vi "Beacon_Filtering_Inter_Beacon_Distance_R1.vi"(0 "Num of Beacons":i8=5, 1 "Inter Beacon\nReal Distance":sgl=3.0, 5 "X in":sgl[](array[numeric]), 7 "Inter Beacon\ndelta Threshold":sgl=1.0, 9 "Y in":sgl[](array[numeric]), 11 "Valid Data\nSets in":bool[](array[boolean])=[TRUE, TRUE, TRUE, TRUE, TRUE]) -> (4 "Beacons Valid - Out":bool[](array[boolean]))   [LabVIEW 2015]
panel:
  in  "Intercept":sgl format="%#_13g"
  in  "Slope":sgl format="%#_13g"
  out "Debug Inter DIstances":sgl[][](array[numeric])
  out "Debug Out\nDistances":sgl[][](array[numeric])
  out "Debug Out\nP/F for each\nanchor":bool[][](array[boolean])
  # "INPUTS"
  # "CONFIG"
  # "OUTPUTS"
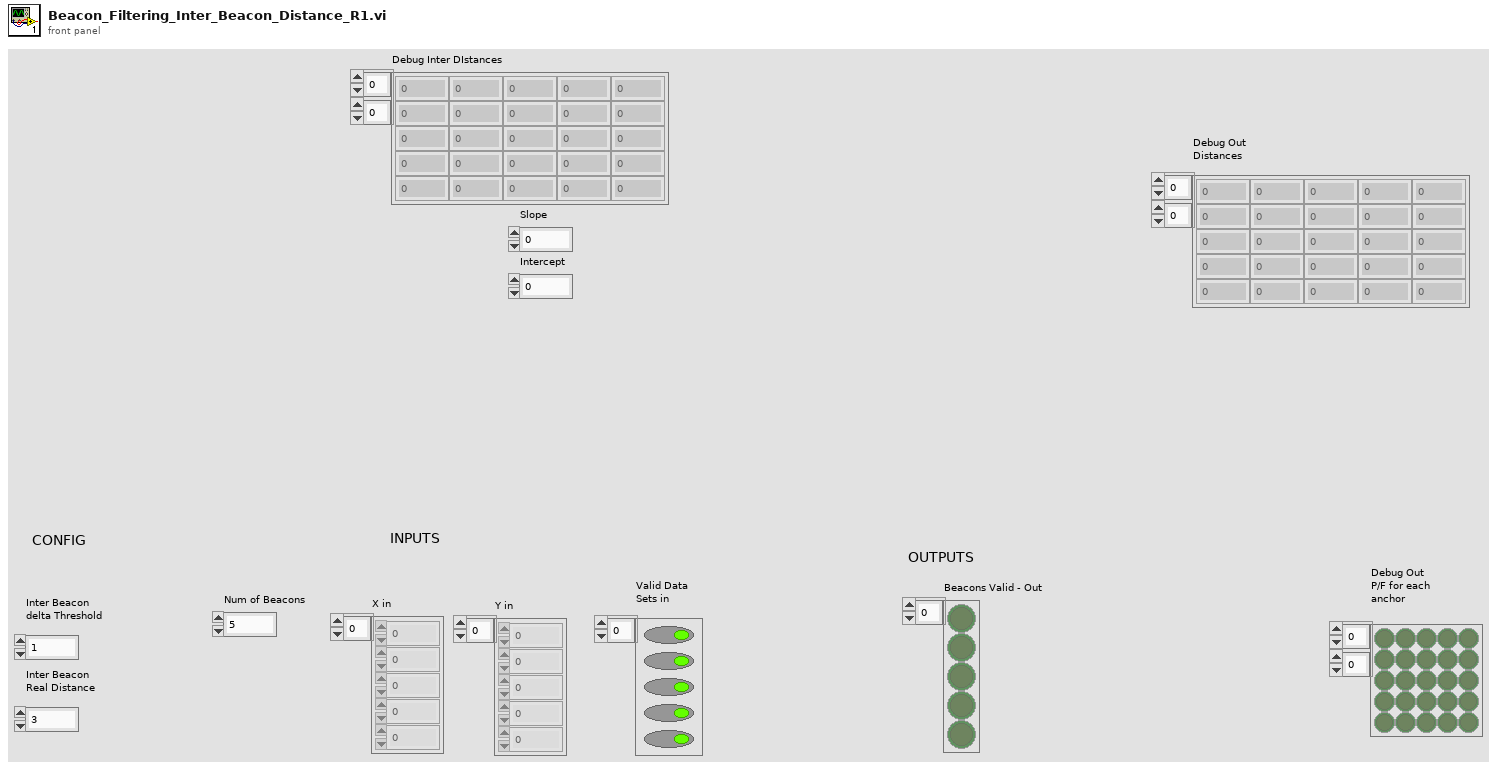
[diagram p1: front panel]
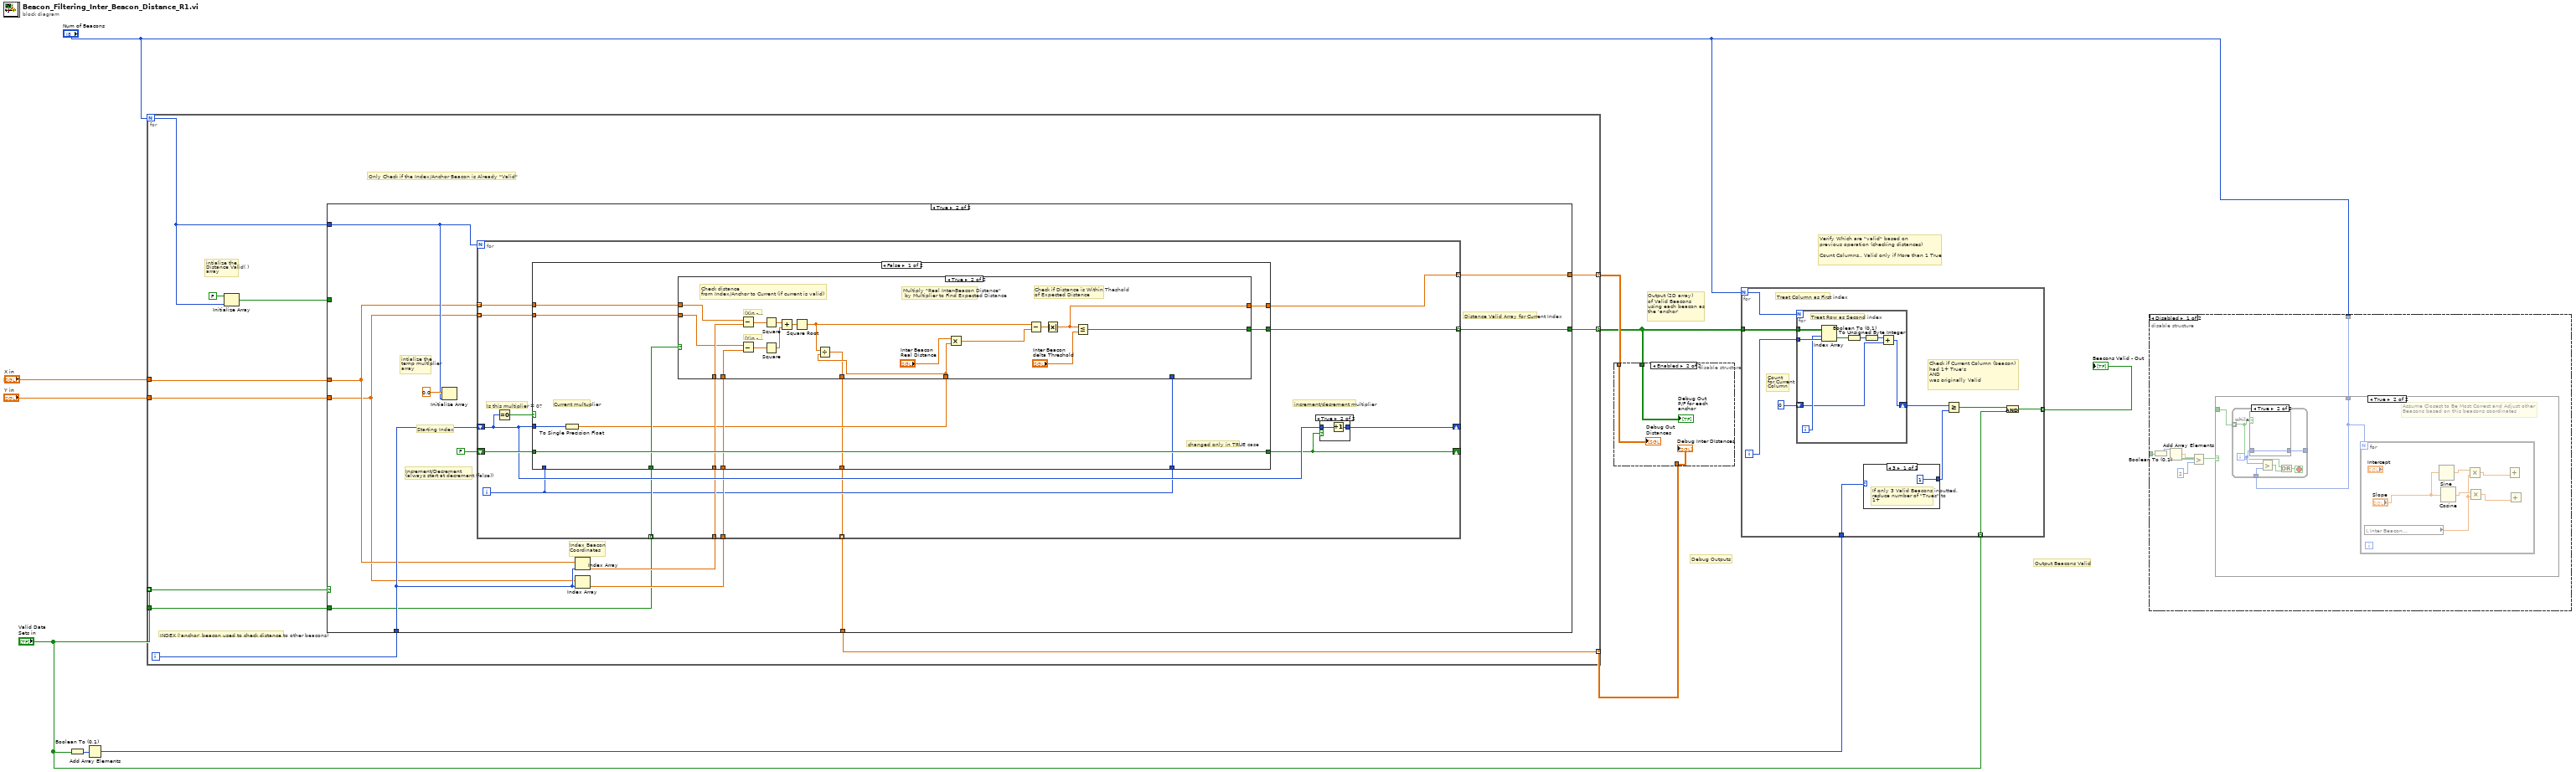
[diagram p0: block diagram]
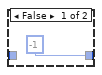
[diagram p3: hidden frame]
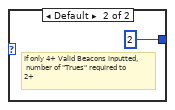
[diagram p6: hidden frame]
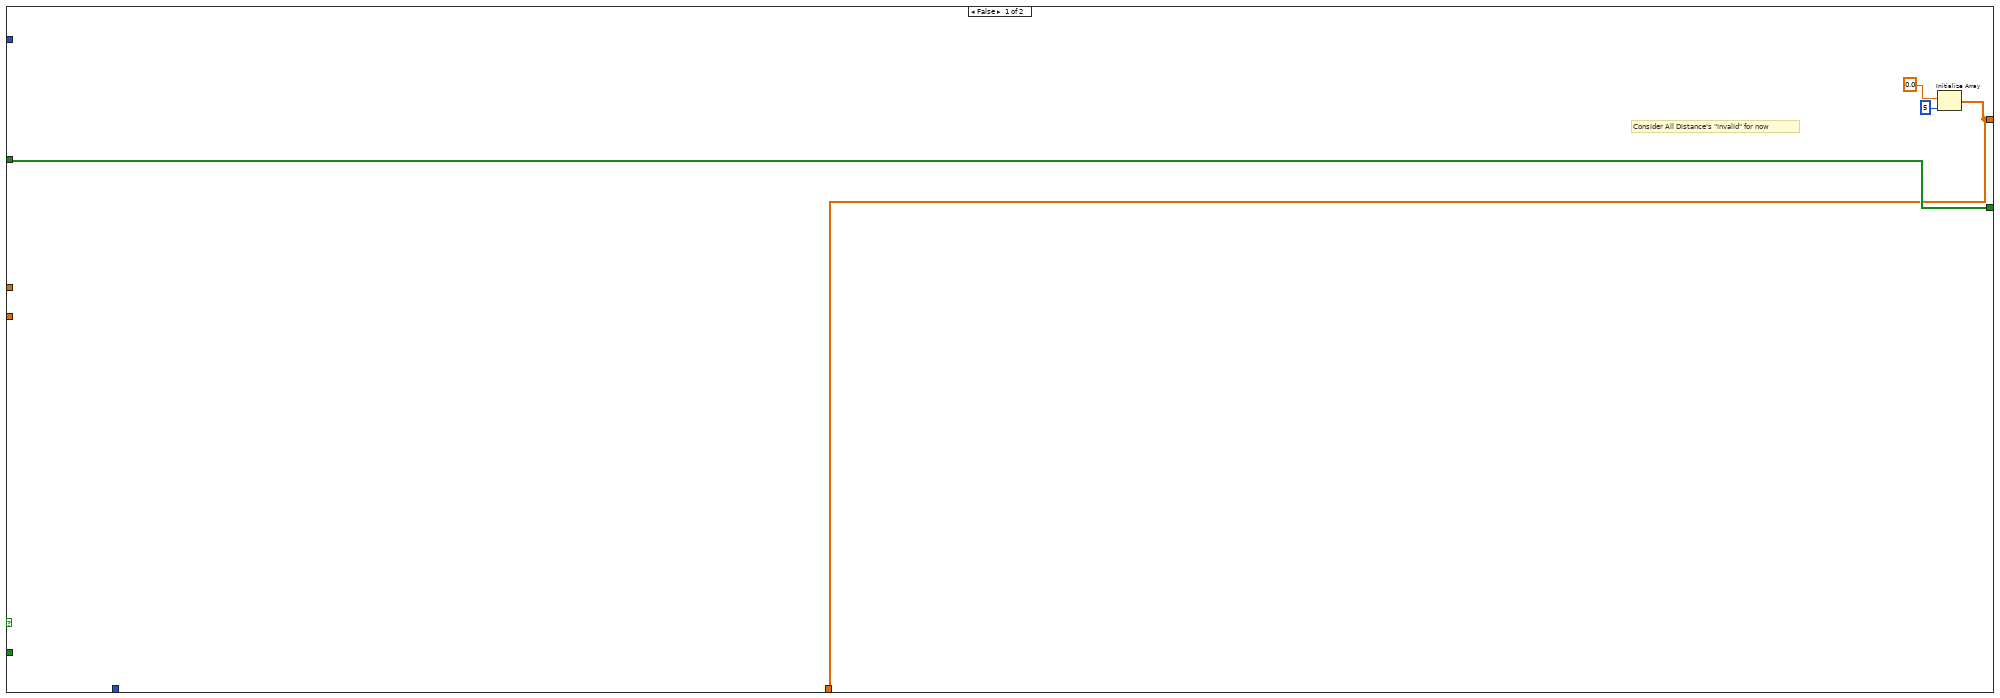
[diagram p7: hidden frame]
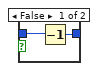
[diagram p8: hidden frame]
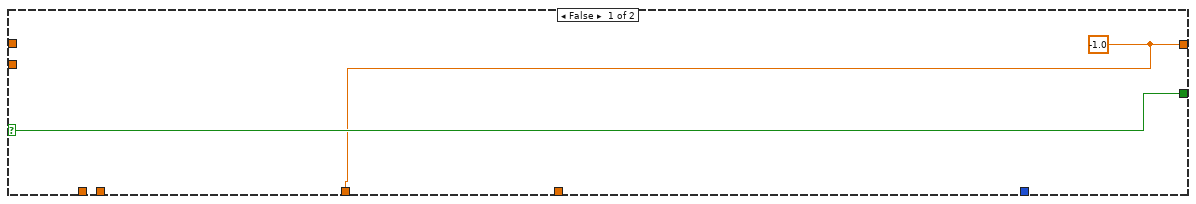
[diagram p9: hidden frame]
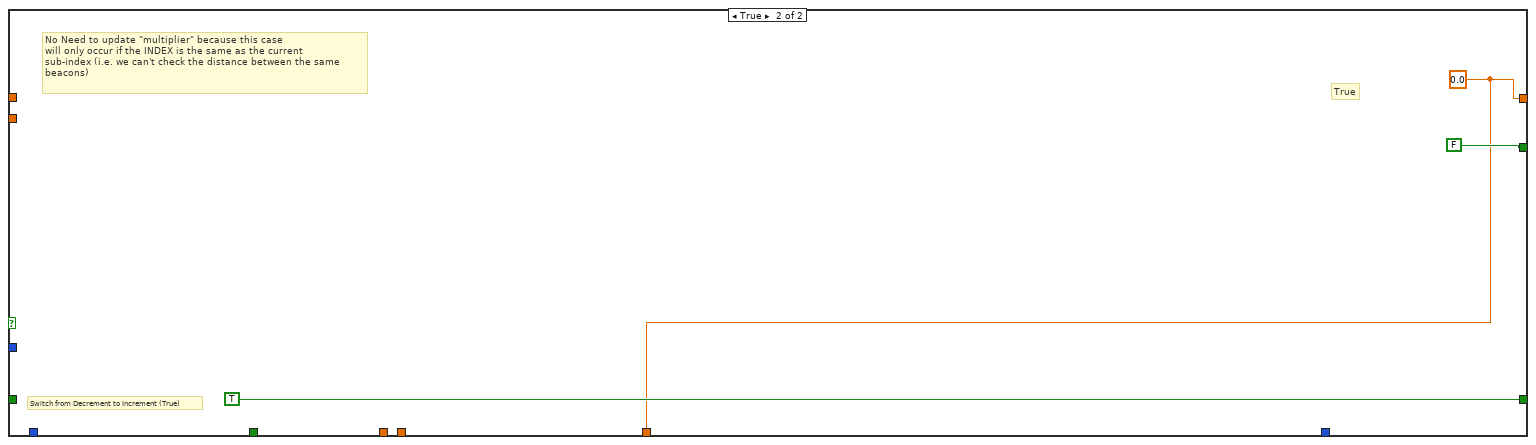
[diagram p10: hidden frame]
diagram:
  # "Debug Outputs"
  # "Output Beacons Valid"
  # "Verify Which are \"valid\" based on \nprevious operation (checking distances)\n\nCount Columns.. Valid only if More than 1 True"
  # "Output (2D array)\nof Valid Beacons\nusing each beacon as\nthe 'anchor'"
  n1 = Boolean To (0,1)(Boolean="Valid Data\nSets in") -> (0, 1=w3:i16[])
  n2 = Add Array Elements(numeric array=w3) -> (sum=w1:i16)
  n3 = for {
    N: "Num of Beacons" -> [w16]
    tunnel: "Valid Data\nSets in" -> [w21] mode=indexing
    tunnel: "X in" -> [w11]
    tunnel: "Y in" -> [w20]
    tunnel: "Valid Data\nSets in" -> [w18]
    tunnel: [w14] -> w4 mode=indexing
    tunnel: [w13] -> w10 mode=indexing
    tunnel: [w12] -> w9 mode=indexing
    i -> [w19]
    # "intialize the \nDistance Valid( )\narray"
    # "INDEX ('anchor' beacon used to check distance to other beacons)"
    # "Only Check if the Index/Anchor Beacon is Already \"Valid\""
    n4 = Initialize Array(FALSE, w16) -> (w15:bool[])
    n5 = case shown="True" w21 {
      tunnel: w11 -> [_ w31]
      tunnel: w20 -> [_ w30]
      tunnel: w19 -> [_ w35]
      tunnel: w16 -> [_ w34]
      tunnel: w18 -> [_ w29]
      tunnel: w15 -> [w25 _]
      tunnel: [w25 w28] -> w14
      tunnel: [w22 w27] -> w13
      tunnel: [w22 w26] -> w12
      frame False {
        # "Consider All Distance's \"invalid\" for now"
        n6 = Initialize Array(sgl 0.0, 5 ("dimension size")) -> (w22:sgl[])
      }
      frame True {
        # "Distance Valid Array for Current Index"
        # "intialize the \ntemp multlplier\narray"
        # "Increment/Decrement\n(always start at decrement (false))"
        # "Starting Index"
        # "Index Beacon\nCoordinates"
        n7 = Initialize Array(sgl 0.0, w34) -> ()  [unwired: 1 out]
        n8 = Index Array(array=w30, index=w35) -> (element=w32:sgl)
        n9 = Index Array(array=w31, index=w35) -> (element=w33:sgl)
        n10 = for {
          N: w34 -> [_]
          shift-right: [w47] -> _
          shift-left: w35 -> [w49]
          shift-right: [w48] -> _
          shift-left: FALSE -> [w50]
          tunnel: w33 -> [w46]
          tunnel: w32 -> [w45]
          tunnel: w31 -> [w44] mode=indexing
          tunnel: w30 -> [w43] mode=indexing
          tunnel: w29 -> [w42] mode=indexing
          tunnel: [w41] -> w28 mode=indexing
          tunnel: [w39] -> w27 mode=indexing
          tunnel: [w38] -> w26 mode=indexing
          i -> [w40]
          # "increment/decrement multiplier"
          # "Is this multiplier = 0?"
          n11 = Equal To 0?(x=w49) -> (x = 0?=w51:bool)
          n12 = case shown="False" w51 {
            tunnel: w49 -> [w67 _]
            tunnel: w40 -> [_ _]
            tunnel: w50 -> [w66 _]
            tunnel: [w66 TRUE] -> w48
            tunnel: w46 -> [w65 _]
            tunnel: w45 -> [w64 _]
            tunnel: w44 -> [w63 _]
            tunnel: w43 -> [w62 _]
            tunnel: w42 -> [w61 _]
            tunnel: [w59 FALSE] -> w41
            tunnel: w40 -> [w58 _]
            tunnel: [w57 w88] -> w39
            tunnel: [w56 w88] -> w38
            frame False {
              # "Current multuplier"
              # "changed only in TRUE case"
              n13 = To Single Precision Float(number=w67) -> (single precision float=w60:sgl)
              n14 = case shown="True" w61 {
                selector: w61 -> [w69 _]
                tunnel: w65 -> [_ w82]
                tunnel: w64 -> [_ w81]
                tunnel: w63 -> [_ w80]
                tunnel: w62 -> [_ w79]
                tunnel: w60 -> [_ w71]
                tunnel: [w69 w74] -> w59
                tunnel: w58 -> [_ _]
                tunnel: [w68 w73] -> w57
                tunnel: [w68 w70] -> w56
                frame False {
                  w68 = sgl -1.0
                }
                frame True {
                  # "Check if Distance is Within Theshold\nof Expected Distance"
                  # "Multiply \"Real Inter-Beacon Distance\"\n by Multiplier to Find Expected Distance"
                  # "(Yin - Y')^2"
                  # "(Xin - X')^2"
                  # "Check distance\nfrom Index/Anchor to Current (if current is valid)"
                  n15 = Subtract(x=w80, y=w82) -> (x-y=w84:sgl)
                  n16 = Subtract(x=w79, y=w81) -> (x-y=w85:sgl)
                  n17 = Square(x=w84) -> (x^2=w86:sgl)
                  n18 = Square(x=w85) -> (x^2=w87:sgl)
                  n19 = Add(x=w86, y=w87) -> (x+y=w83:sgl)
                  n20 = Square Root(x=w83) -> (sqrt(x)=w72:sgl)
                  n21 = Divide(x=w72, y=w71) -> (x/y=w70:sgl)
                  n22 = Multiply(x="Inter Beacon\nReal Distance", y=w71) -> (x*y=w77:sgl)
                  n23 = Subtract(x=w72, y=w77) -> (x-y=w76:sgl)
                  n24 = Absolute Value(x=w76) -> (abs(x)=w73:sgl)
                  n25 = Less Or Equal?(x=w73, y="Inter Beacon\ndelta Threshold") -> (x <= y?=w74:bool)
                }
              }
            }
            frame True {
              w88 = sgl 0.0
              # "True"
              # "Switch from Decrement to Increment (True)"
              # "No Need to update \"multiplier\" because this case\nwill only occur if the INDEX is the same as the current \nsub-index (i.e. we can't check the distance between the same\nbeacons)"
            }
          }
          n26 = case shown="True" w48 {
            tunnel: w49 -> [w53 w55]
            tunnel: [w52 w54] -> w47
            frame False {
              n27 = Decrement(x=w53) -> (x-1=w52:i32)
            }
            frame True {
              n28 = Increment(x=w55) -> (x+1=w54:i32)
            }
          }
        }
      }
    }
  }
  n29 = disable-structure shown="Enabled" {
    disable-tunnel: w4 -> [_ w92]
    disable-tunnel: w10 -> [_ w93]
    disable-tunnel: w9 -> [_ w91]
    frame Disabled {
    }
    frame Enabled {
      "Debug Out\nP/F for each\nanchor" <- w92
      "Debug Out\nDistances" <- w93
      "Debug Inter DIstances" <- w91
    }
  }
  n30 = for {
    N: "Num of Beacons" -> [w95]
    tunnel: w4 -> [w103]
    tunnel: "Valid Data\nSets in" -> [w96] mode=indexing
    tunnel: [w97] -> w6 mode=indexing
    tunnel: w1 -> [w94]
    i -> [w102]
    # "Check if Current Column (beacon)\nhad 1+ True's \nAND \nwas originally Valid"
    # "Count\nfor Current\nColumn"
    # "Treat Column as First index"
    n31 = for {
      N: w95 -> [_]
      tunnel: w103 -> [w113]
      tunnel: w102 -> [w112]
      shift-right: [w106] -> w99
      shift-left: u8 0 -> [w108]
      i -> [w111]
      # "Treat Row as Second index"
      n32 = Index Array(array=w113, index (row)=w111, index (col)=w112) -> (element=w110:bool)
      n33 = Boolean To (0,1)(Boolean=w110) -> (0, 1=w109:i16)
      n34 = To Unsigned Byte Integer(number=w109) -> (unsigned 8bit integer=w107:u8)
      n35 = Add(x=w107, y=w108) -> (x+y=w106:u8)
    }
    n36 = case shown="3" w94 {
      tunnel: [u8 1 u8 2] -> w100
      frame 3 {
        # "If only 3 Valid Beacons inputted,\nreduce number of \"Trues\" to\n1+"
      }
      frame Default {
        # "If only 4+ Valid Beacons inputted,\n number of \"Trues\" required to\n2+"
      }
    }
    n37 = Greater Or Equal?(x=w99, y=w100) -> (x >= y?=w98:bool)
    n38 = And(x=w98, y=w96) -> (x .and. y?=w97:bool)
  }
  "Beacons Valid - Out" <- w6
  n39 = disable-structure shown="Disabled" {
    disable-tunnel: _ -> [w115 _]
    disable-tunnel: "Num of Beacons" -> [w114 _]
    frame Disabled {
      n40 = Boolean To (0,1)(Boolean=w115) -> (0, 1=w116:i16)
      n41 = Add Array Elements(numeric array=w116) -> (sum=w117:dbl)
      n42 = Greater?(x=w117, y=u8 2) -> (0:w118:bool)
      n43 = case shown="True" w118 {
        tunnel: _ -> [_ w121]
        tunnel: w114 -> [_ w120]
        frame False {
        }
        frame True {
          # "Assume Closest to Be Most Correct and Adjust other\nBeacons based on this beacons coordinates"
          n44 = while {
            tunnel: w121 -> [w130] mode=indexing
            tunnel: [w132] -> _
            tunnel: w120 -> [w128]
            i -> [w133]
            stop <- w129 stop-if-true
            n45 = case shown="True" w130 {
              tunnel: w133 -> [_ w135]
              tunnel: [-1 w135] -> w132
              frame False {
              }
              frame True {
              }
            }
            n46 = Greater?(x=w133, y=w128) -> (0:w131:bool)
            n47 = Or(x=w130, y=w131) -> (x .or. y?=w129:bool)
          }
          n48 = for {
            N: w120 -> [_]
            n49 = local read "Inter Beacon\nReal Distance"() -> (w124:sgl)
            n50 = Sine(x="Slope") -> (sin(x)=w126:sgl)
            n51 = Cosine(x="Slope") -> (cos(x)=w125:sgl)
            n52 = Multiply(x=w126, y=w124) -> (x*y=w122:sgl)
            n53 = Multiply(x=w125, y=w124) -> (x*y=w123:sgl)
            n54 = Add(y=w122) -> ()  [unwired: 1 in, 1 out]
            n55 = Add(y=w123) -> ()  [unwired: 1 in, 1 out]
          }
        }
      }
    }
    frame Enabled {
    }
  }
